vi "Byte Buffer.Mapping.Create (Block Descriptor).vi"(8 "error in (no error)":errorcluster, 9 "data type":T3, 10 "buffer offset":i32, 11 "Channel Block Descriptor":T1) -> (0 "error out":errorcluster, 2 "new buffer offset":i32, 3 "mapping":T4)   [LabVIEW 2016, in "VeriStand Data.lvlib" / "Byte Buffer.lvclass"]
uses:
  Byte Buffer.lvclass
  Byte Buffer.Mapping.ctl
  Typedefs/Typedefs.Data Types.ctl
  Typedefs/Typedefs.Block Descriptor.Channel Block.ctl
  Typedefs/Typedefs.Block Descriptor.ctl
  Utilities/Utilities.Sizeof.Scalar.vi
  VeriStand Data.lvlib
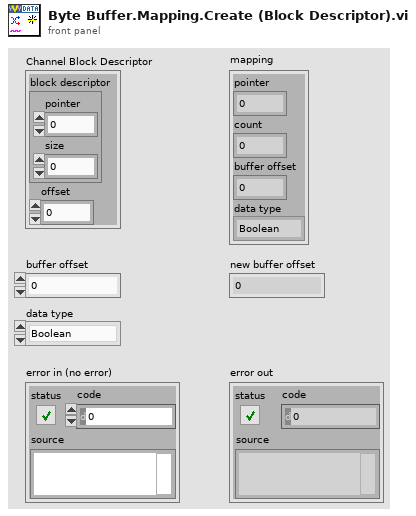
[diagram p1: front panel]
types:
  T1 = typedef "VeriStand Data.lvlib/Typedefs.Block Descriptor.Channel Block.ctl" = cluster{"block descriptor":T2, "offset":u64}
  T2 = typedef "VeriStand Data.lvlib/Typedefs.Block Descriptor.ctl" = cluster{"pointer":u64, "size":u64}
  T3 = typedef "VeriStand Data.lvlib/Typedefs.Data Types.ctl" = enum16{"Boolean", "Single", "Double", "I8", "I16", "I32", "I64", "U8", "U16", "U32", "U64"}
  T4 = typedef "VeriStand Data.lvlib/Byte Buffer.lvclass/Byte Buffer.Mapping.ctl" = cluster{"pointer":u64, "count":i32, "buffer offset":i32, "data type":T3}
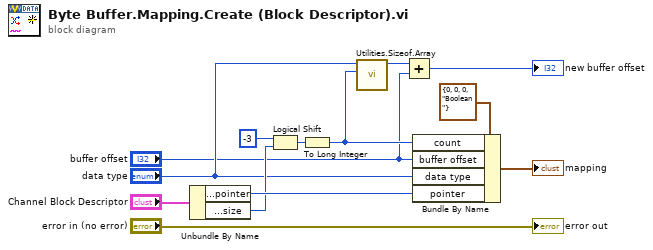
[diagram p0: block diagram]
diagram:
  n1 = Unbundle By Name("Channel Block Descriptor") -> ("block descriptor.pointer"=w11:u64, "block descriptor.size"=w9:u64)
  n2 = Logical Shift(y=i16 -3, x=w9) -> (x << y=w10:u64)
  n3 = To Long Integer(number=w10) -> (32bit integer=w2:i32)
  n4 = call "Utilities.Sizeof.Array.vi"("count"=w2, "data type"="data type") -> ("size"=w5:i32)  [unwired: 9 in]
  n5 = Add(x=w5, y="buffer offset") -> (x+y=→"new buffer offset":i32)
  n6 = Bundle By Name(cluster=T4 {"pointer"=0, "count"=0, "buffer offset"=0, "data type"=enum."Boolean"} ("mapping"), "count"=w2, "buffer offset"="buffer offset", "data type"="data type", "pointer"=w11) -> (→"mapping":T4)
  "error out" <- "error in (no error)"
